vi "Check Error.vi"(6 "Case":string="Idle", 7 "Filtered Error Codes":i32[](array[numeric])=[91, -314302], 8 "error in":errorcluster) -> (0 "error out":errorcluster, 3 "Error?":bool)   [LabVIEW 2019]
doc: "This VI is part of the QDMH template. It checks the error code to see if a non-filtered error has occured. If it has, it will place the Error case on the queue and add the pertinent information to the data variant. It will also clear the error.\n\nAAL 9/09"
uses:
  Support/User Event/User Evnet AE data.ctl
  Support/User Event/User Events AE Control.ctl
  Support/User Event/User Event.lvlib
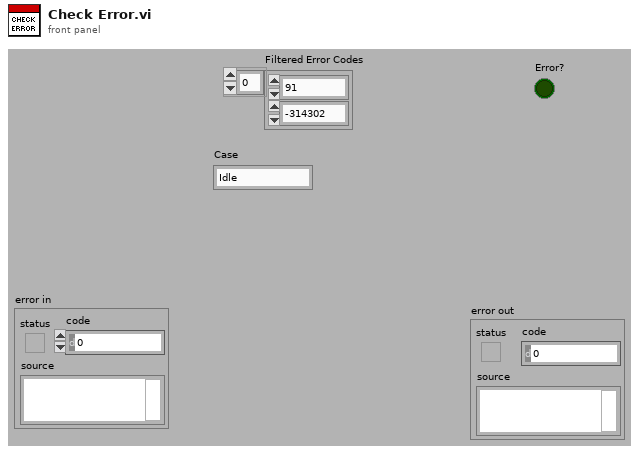
[diagram p1: front panel]
types:
  T1 = typedef "User Event.lvlib/User Events AE Control.ctl" = enum16{"Create", "Get", "Generate", "Destroy"}
  T2 = typedef "User Event.lvlib/User Evnet AE data.ctl" = cluster{"Data":variant, "Message":string}
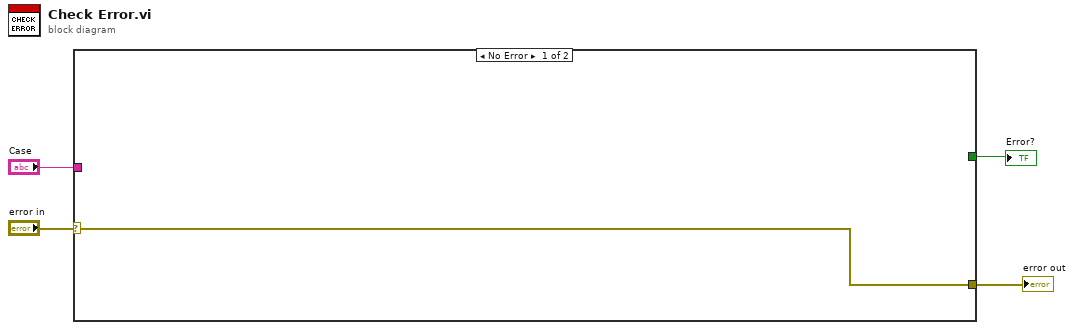
[diagram p0: block diagram]
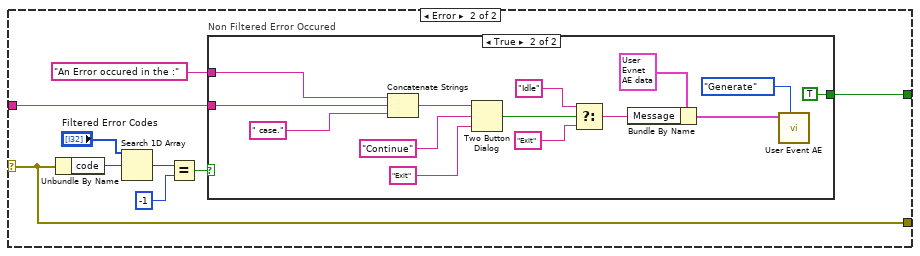
[diagram p2: hidden frame]
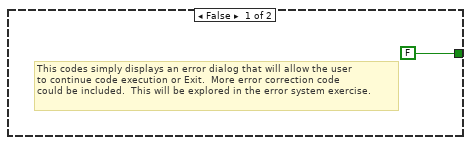
[diagram p3: hidden frame]
diagram:
  n1 = case shown="No Error" "error in" {
    selector: "error in" -> [w5 w7]
    tunnel: [w5 w7] -> w4
    tunnel: "Case" -> [_ w14]
    tunnel: [_ w6] -> w1
    frame No Error {
    }
    frame Error {
      n2 = Unbundle By Name(w7) -> ("code"=w13:i32)
      n3 = Search 1D Array(1D array="Filtered Error Codes", element=w13) -> (index of element=w11:i32)  [unwired: 1 out]
      n4 = Equal?(x=w11, y=-1) -> (x = y?=w9:bool)
      n5 = case "Non Filtered Error Occured" shown="True" w9 {
        tunnel: w14 -> [_ w21]
        tunnel: "An Error occured in the :" ("string") -> [_ w17]
        tunnel: [FALSE ("Error?") TRUE ("Error?")] -> w6
        frame False {
          # "This codes simply displays an error dialog that will allow the user\nto continue code execution or Exit.  More error correction code\ncould be included.  This will be explored in the error system exercise."
        }
        frame True {
          n6 = Concatenate Strings(w17, w21, " case." ("string")) -> (w27:string)
          n7 = Two Button Dialog(message=w27, 1:"Exit" ("F button name (\"Cancel\")"), 2:"Continue" ("T button name (\"OK\")")) -> (T button?=w25:bool)
          n8 = Select(t="Idle" ("F button name (\"Cancel\")"), s=w25, f="Exit" ("F button name (\"Cancel\")")) -> (s? t:f=w29:string)
          n9 = Bundle By Name(cluster=T2 {"Data"=variant, "Message"=""} ("event data"), "Message"=w29) -> (w19:T2)
          n10 = call "User Event AE.vi"("Control"=User_Events_AE_Control."Generate", "event data"=w19) -> ()  [unwired: 8 in, 2 out]
        }
      }
    }
  }
  "error out" <- w4
  "Error?" <- w1
